vi "translateDigitalInputs.vi"(0 "SingleAxisController in":refnum<class "_SingleAxisController.lvclass">, 2 "di_value (in)":u32, 5 "error in (no error)":errorcluster) -> (14 "SingleAxisController out":refnum<class "_SingleAxisController.lvclass">, 16 "dig_in_value (out)":u32, 17 "dig_in_items (out)":T1[](array[typedef]), 19 "error out":errorcluster)   [LabVIEW 2013, in "classes.lvlib" / "_SingleAxisController.lvclass"]
doc: "Translates the Digital Inputs for Single-Axis Controllers\n\nProduced By:\n\n<B>Kod Integrations, LLC</B>\n4835 Marianne Drive\nMount Airy, MD 21771\nhttp://www.kodintegrations.com\nemail: info@kodintegrations.com\nphone: (240) 687-1288"
uses:
  _SingleAxisController.lvclass
  digital_input_item.ctl
  digital_input.ctl
  common.lvlib
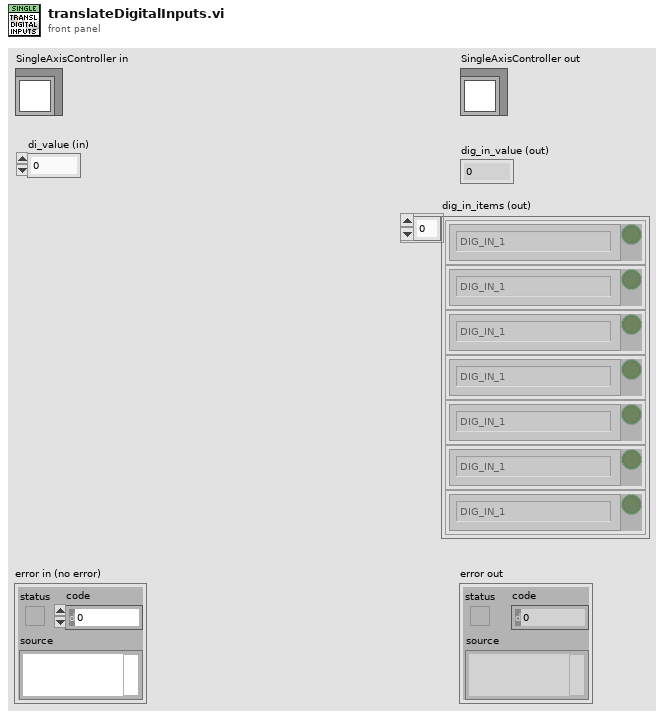
[diagram p1: front panel]
types:
  T1 = typedef "common.lvlib/digital_input_item.ctl" = cluster{"item":T2, "status":bool}
  T2 = typedef "common.lvlib/digital_input.ctl" = enum16{"DIG_IN_1", "DIG_IN_2", "DIG_IN_3", "DIG_IN_4", "DIG_IN_5", "DIG_IN_6", "DIG_IN_7", "DIG_IN_8", "NEG_LIMIT", "HOME", "POS_LIMIT"}
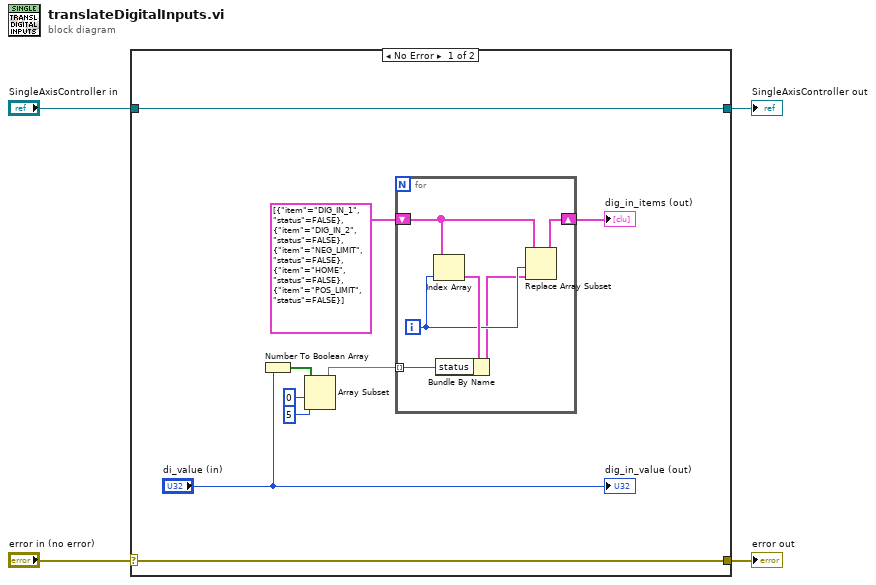
[diagram p0: block diagram]
diagram:
  n1 = case shown="No Error" "error in (no error)" {
    selector: "error in (no error)" -> [w12 w21]
    tunnel: [w12 w21] -> w3
    tunnel: [w13 w20] -> w1
    tunnel: "SingleAxisController in" -> [w13 w20]
    frame No Error {
      n2 = Number To Boolean Array(number="di_value (in)") -> (Boolean array=w10:bool[])
      n3 = Array Subset(array=w10, index=0, length=5) -> (w7:bool[])
      n4 = for {
        shift-right: [w14] -> w6
        shift-left: T1[] [{"item"=enum."DIG_IN_1", "status"=FALSE}, {"item"=enum."DIG_IN_2", "status"=FALSE}, {"item"=enum."NEG_LIMIT", "status"=FALSE}, {"item"=enum."HOME", "status"=FALSE}, {"item"=enum."POS_LIMIT", "status"=FALSE}] ("polarity_items (in)") -> [w17]
        tunnel: w7 -> [w18] mode=indexing
        i -> [w16]
        n5 = Index Array(array=w17, index=w16) -> (element=w19:T1)
        n6 = Bundle By Name(cluster=w19, "status"=w18) -> (w15:T1)
        n7 = Replace Array Subset(array=w17, new element=w15, index=w16) -> (w14:T1[])
      }
      "dig_in_items (out)" <- w6
      "dig_in_value (out)" <- "di_value (in)"
    }
    frame Error {
    }
  }
  "error out" <- w3
  "SingleAxisController out" <- w1
